vi "Initialize Fixed-Point Configuration.vi"(8 "error in (no error)":errorcluster, 11 "Numeric Data Type in":refnum<class "Numeric Data Type.lvclass">) -> (0 "error out":errorcluster, 3 "Numeric Data Type (dup)":refnum<class "Numeric Data Type.lvclass">)   [LabVIEW 2018, in "Numeric Data Type.lvclass"]
uses:
  Numeric Data Type.lvclass
  Representation Enum.ctl
  Numeric Data Type.lvclass/Numeric Data Type.ctl
  <vilib>/fxp/FXPxcontrol/FXP.xctl
  Reference Fixed-Point Configuration.vi
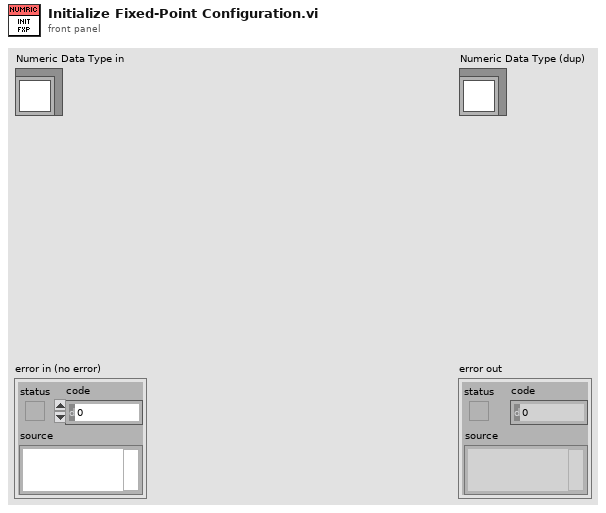
[diagram p1: front panel]
types:
  T1 = enum8{"Enabled", "Disabled", "Disabled and Grayed Out"}
  T2 = typedef "Numeric Data Type.lvclass/Representation Enum.ctl" = enum16{"Extended (EXT)", "Double (DBL)", "Single (SGL)", "Fixed-Point (FXP)", "Quad Integer (I64)", "Long Integer (I32)", "Word Integer (I16)", "Byte Integer (I8)", "Unsigned Quad (U64)", "Unsigned Long (U32)", "Unsigned Word (U16)", "Unsigned Byte (U8)", "Complex Extended (CXT)", "Complex Double (CDB)", "Complex Single (CSG)"}
  T3 = typedef "Numeric Data Type.lvclass/Fixed-Point Value.ctl" = cluster{"Encoding":cluster{"Signed":bool, "Word Length":u32, "Integer Word Length":i32}, "Range":cluster{"Range Min":dbl, "Range Max":dbl, "Delta":dbl}}
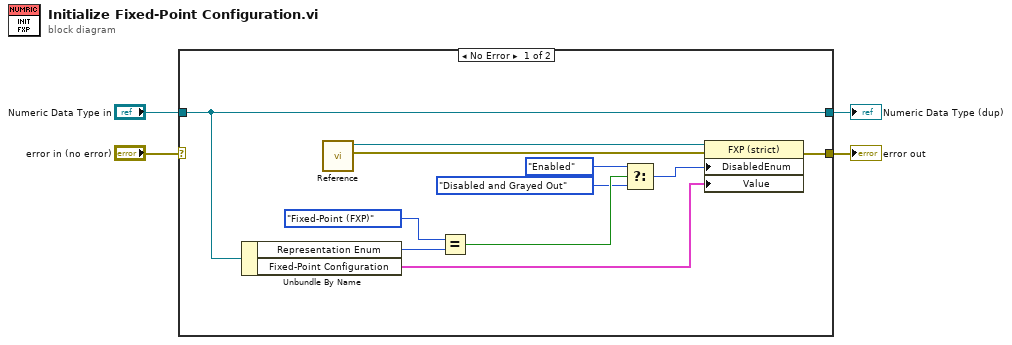
[diagram p0: block diagram]
diagram:
  n1 = case shown="No Error" "error in (no error)" {
    selector: "error in (no error)" -> [_ w17]
    tunnel: [w5 w17] -> w3
    tunnel: [w15 w16] -> w1
    tunnel: "Numeric Data Type in" -> [w15 w16]
    frame No Error {
      n2 = Unbundle By Name(w15) -> ("Representation Enum"=w9:T2, "Fixed-Point Configuration"=w13:T3)
      n3 = call-poly "Reference.vi"() -> ("error out"=w12:errorcluster, "Fixed-Point Configuration"=w14:refnum<vi>)  [unwired: 10 in]
      n4 = Equal?(x=Representation_Enum."Fixed-Point (FXP)", y=w9) -> (x = y?=w7:bool)
      n5 = Select(t=T1."Enabled" ("Disabled"), s=w7, f=T1."Disabled and Grayed Out" ("Disabled")) -> (s? t:f=w10:T1)
      n6 = property class="FXP (strict)"(reference=w14, error in=w12, "DisabledEnum"=w10, "Value"=w13) -> (error out=w5:errorcluster)  [unwired: 1 out]
    }
    frame Error {
    }
  }
  "error out" <- w3
  "Numeric Data Type (dup)" <- w1
